vi "Autonomous Independent.vi"   [LabVIEW 2017]
doc: "This VI is called when autonomous begins, and will automatically be terminated when autonomous ends. You can carry out timed or sensor driven robot movement independently without needing to return to the caller."
uses:
  AutonActions.ctl
  WristPositions.ctl
  <vilib>/Rock Robotics/Network Tables/NT Write String.vi
  <vilib>/Rock Robotics/Network Tables/NT Read Number.vi
types:
  T1 = cluster{"TrgtCounts":i32, "CurrCounts":dbl, "SlowRng":dbl}
  T2 = cluster{"Heading":dbl, "Initial":dbl, "Range":dbl, "GyroSens":dbl}
  T3 = typedef "AutonActions.ctl" = enum16{"Initialize", "Stop", "Reset", "StraightForward", "StraightBack", "SolenoidControl", "TurnLeft90", "TurnRight90", "TurnLeft45", "TurnRight45", "PivotLeft90", "PivotRight90", "PivotLeft45", "PivotRight45", "PivotLeft30", "PivotRight30", "StraightForwardTime", "Release", "Shoot", "Wrist", "GripperToggle", "ElevUp", "ElevDown", "Pause", ""}
  T4 = typedef "WristPositions.ctl" = enum16{"MostDown", "AllDown", "MostUp", "AllUp"}
  T5 = cluster{"Action":T3, "DriveEncCnts":i32, "Accel?":bool, "Decel?":bool, "ElevEncCnts":i32, "Action2":T3, "Action2Trigger":i32, "WristPositions":T4, "SlowRng":dbl}[]
  T6 = cluster{"Action":T3, "DriveEncCnts":i32, "Accel?":bool, "Decel?":bool, "ElevEncCnts":i32, "Action2":T3, "Action2Trigger":i32, "WristPositions":T4, "SlowRng":dbl}
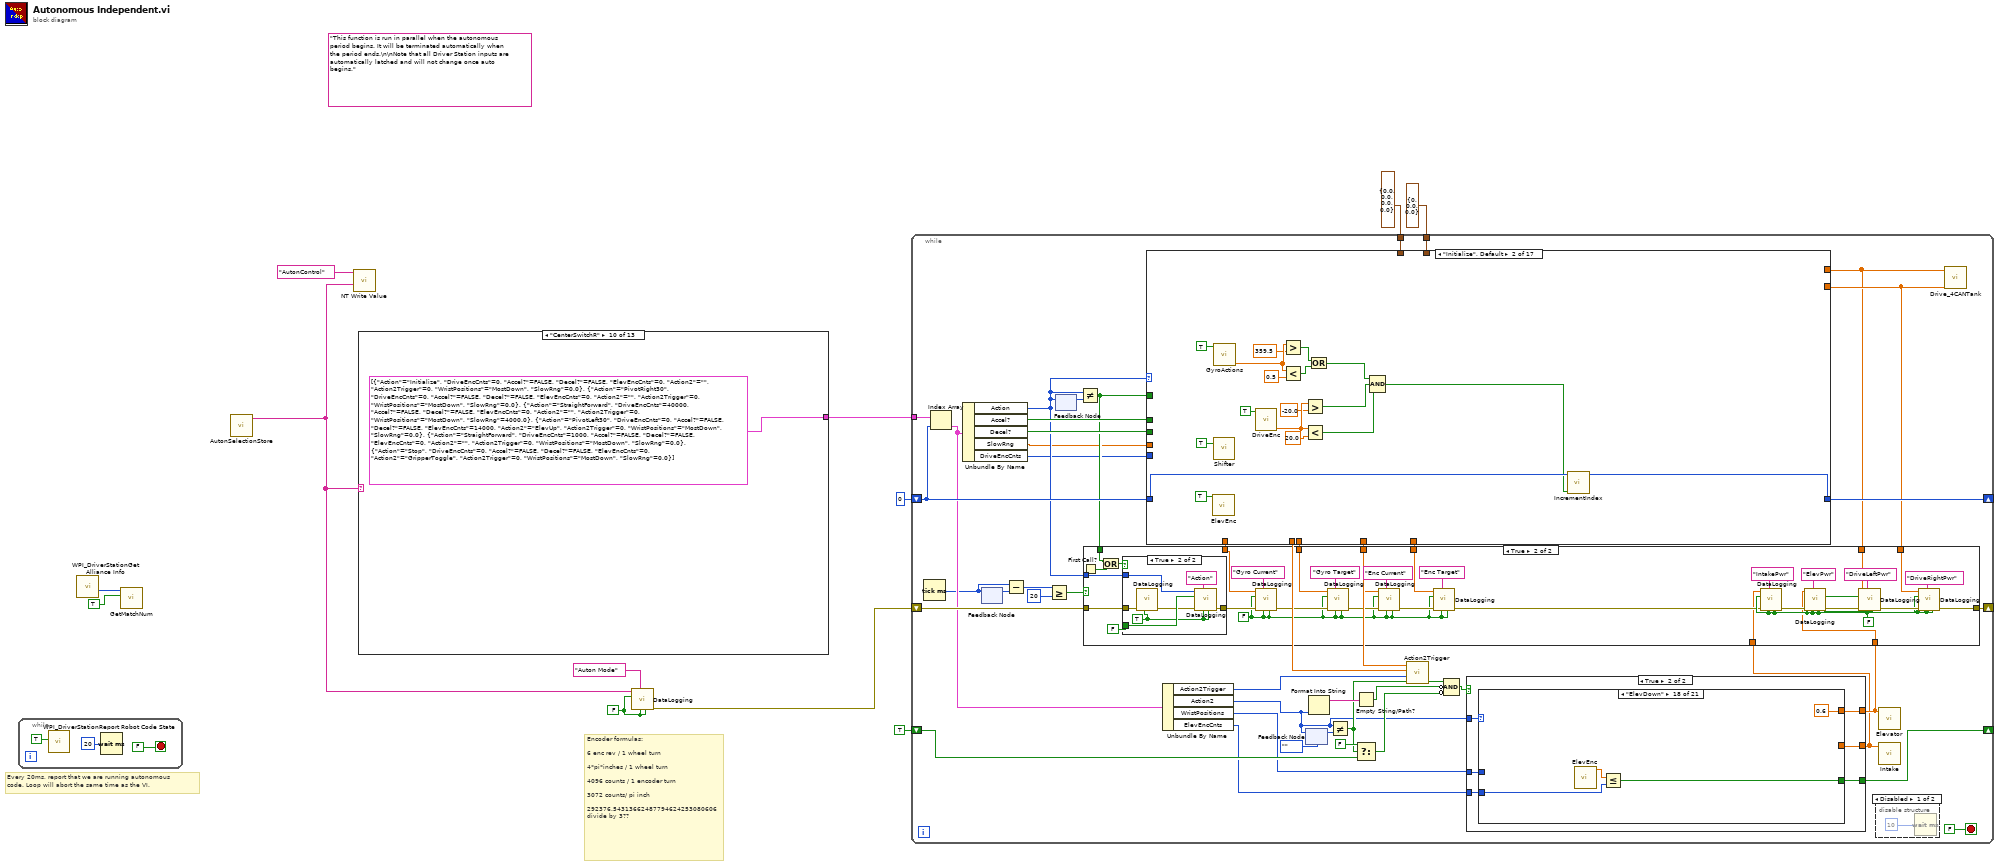
[diagram p0: block diagram]
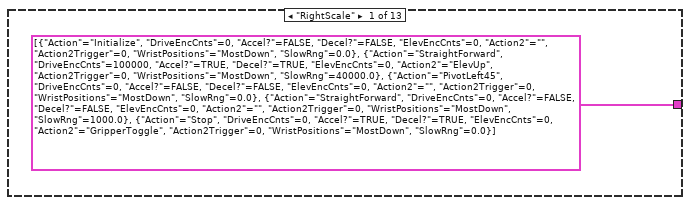
[diagram p2: hidden frame]
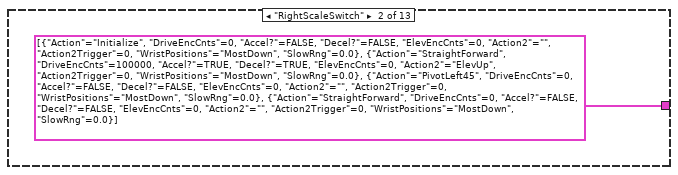
[diagram p3: hidden frame]
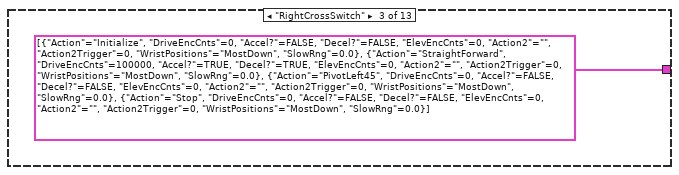
[diagram p4: hidden frame]
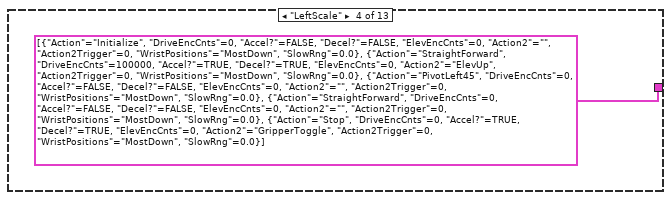
[diagram p5: hidden frame]
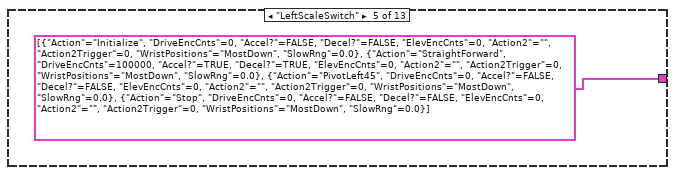
[diagram p6: hidden frame]
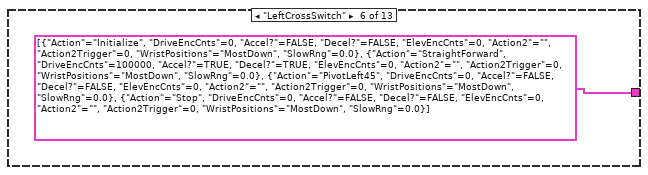
[diagram p7: hidden frame]
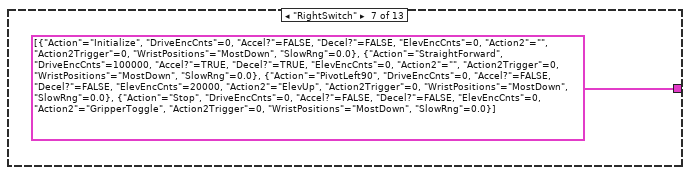
[diagram p8: hidden frame]
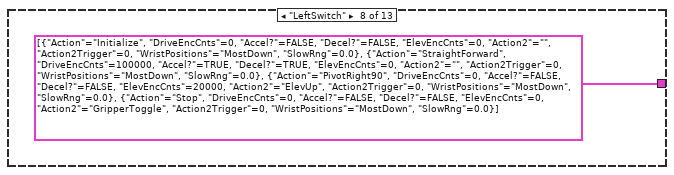
[diagram p9: hidden frame]
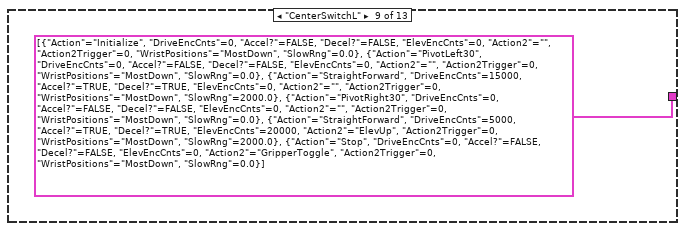
[diagram p10: hidden frame]
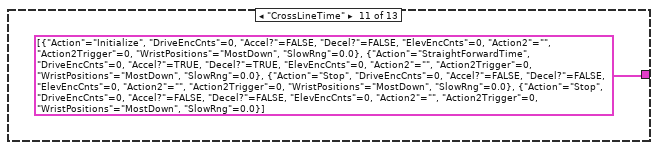
[diagram p11: hidden frame]
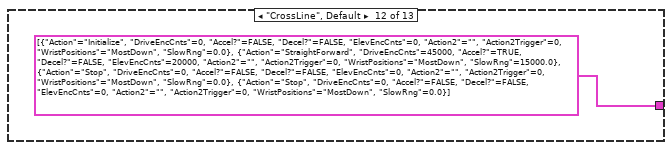
[diagram p12: hidden frame]
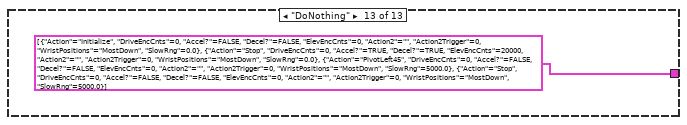
[diagram p13: hidden frame]
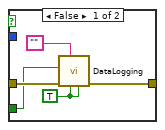
[diagram p15: hidden frame]
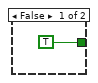
[diagram p16: hidden frame]
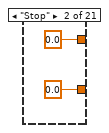
[diagram p18: hidden frame]
diagram:
  w7 = FALSE ("WriteToFile?")
  (unwired) "This function is run in parallel when the autonomous period begins. It will be terminated automatically when the period ends.\n\nNote that all Driver Station inputs are automatically latched and will not change once auto begins."
  # "Encoder formulas:\n\n6 enc rev / 1 wheel turn\n\n4*pi*inches / 1 wheel turn \n\n4096 counts / 1 encoder turn\n\n3072 counts/ pi inch\n\n292376.54313662487794624253080606\ndivide by 3??"
  # "Every 20ms, report that we are running autonomous\ncode. Loop will abort the same time as the VI."
  n1 = while {
    stop <- FALSE stop-if-true
    n2 = call <vilib>:"WPI_DriverStationReport Robot Code State.vi"("Autonomous"=TRUE) -> ()  [unwired: 10 in, 1 out]
    n3 = Wait (ms)(milliseconds to wait=u32 20) -> ()  [unwired: 1 out]
  }
  n4 = call <vilib>:"WPI_DriverStationGet Alliance Info.vi"() -> ("Match Number"=w6:u16)  [unwired: 11 out]
  n5 = call "GetMatchNum.vi"("Update?"=TRUE, "MatchNumberIn"=w6) -> ()  [unwired: 6 in, 1 out]
  n6 = call "AutonSelectionStore.vi"() -> ("AutonSelectionOut"=w1:string)  [unwired: 11 in]
  n7 = call-poly <vilib>:"NT Write Value.vi"("String"=w1, "Name"="AutonControl") -> ()  [unwired: 9 in, 1 out]
  n8 = case shown="\"CenterSwitchR\"" w1 {
    tunnel: [T5 [{"Action"=enum."Initialize", "DriveEncCnts"=0, "Accel?"=FALSE, "Decel?"=FALSE, "ElevEncCnts"=0, "Action2"=enum."", "Action2Trigger"=0, "WristPositions"=enum."MostDown", "SlowRng"=0.0}, {"Action"=enum."StraightForward", "DriveEncCnts"=100000, "Accel?"=TRUE, "Decel?"=TRUE, "ElevEncCnts"=0, "Action2"=enum."ElevUp", "Action2Trigger"=0, "WristPositions"=enum."MostDown", "SlowRng"=40000.0}, {"Action"=enum."PivotLeft45", "DriveEncCnts"=0, "Accel?"=FALSE, "Decel?"=FALSE, "ElevEncCnts"=0, "Action2"=enum."", "Action2Trigger"=0, "WristPositions"=enum."MostDown", "SlowRng"=0.0}, {"Action"=enum."StraightForward", "DriveEncCnts"=0, "Accel?"=FALSE, "Decel?"=FALSE, "ElevEncCnts"=0, "Action2"=enum."", "Action2Trigger"=0, "WristPositions"=enum."MostDown", "SlowRng"=1000.0}, {"Action"=enum."Stop", "DriveEncCnts"=0, "Accel?"=TRUE, "Decel?"=TRUE, "ElevEncCnts"=0, "Action2"=enum."GripperToggle", "Action2Trigger"=0, "WristPositions"=enum."MostDown", "SlowRng"=0.0}] T5 [{"Action"=enum."Initialize", "DriveEncCnts"=0, "Accel?"=FALSE, "Decel?"=FALSE, "ElevEncCnts"=0, "Action2"=enum."", "Action2Trigger"=0, "WristPositions"=enum."MostDown", "SlowRng"=0.0}, {"Action"=enum."StraightForward", "DriveEncCnts"=100000, "Accel?"=TRUE, "Decel?"=TRUE, "ElevEncCnts"=0, "Action2"=enum."ElevUp", "Action2Trigger"=0, "WristPositions"=enum."MostDown", "SlowRng"=0.0}, {"Action"=enum."PivotLeft45", "DriveEncCnts"=0, "Accel?"=FALSE, "Decel?"=FALSE, "ElevEncCnts"=0, "Action2"=enum."", "Action2Trigger"=0, "WristPositions"=enum."MostDown", "SlowRng"=0.0}, {"Action"=enum."StraightForward", "DriveEncCnts"=0, "Accel?"=FALSE, "Decel?"=FALSE, "ElevEncCnts"=0, "Action2"=enum."", "Action2Trigger"=0, "WristPositions"=enum."MostDown", "SlowRng"=0.0}] T5 [{"Action"=enum."Initialize", "DriveEncCnts"=0, "Accel?"=FALSE, "Decel?"=FALSE, "ElevEncCnts"=0, "Action2"=enum."", "Action2Trigger"=0, "WristPositions"=enum."MostDown", "SlowRng"=0.0}, {"Action"=enum."StraightForward", "DriveEncCnts"=100000, "Accel?"=TRUE, "Decel?"=TRUE, "ElevEncCnts"=0, "Action2"=enum."", "Action2Trigger"=0, "WristPositions"=enum."MostDown", "SlowRng"=0.0}, {"Action"=enum."PivotLeft45", "DriveEncCnts"=0, "Accel?"=FALSE, "Decel?"=FALSE, "ElevEncCnts"=0, "Action2"=enum."", "Action2Trigger"=0, "WristPositions"=enum."MostDown", "SlowRng"=0.0}, {"Action"=enum."Stop", "DriveEncCnts"=0, "Accel?"=FALSE, "Decel?"=FALSE, "ElevEncCnts"=0, "Action2"=enum."", "Action2Trigger"=0, "WristPositions"=enum."MostDown", "SlowRng"=0.0}] T5 [{"Action"=enum."Initialize", "DriveEncCnts"=0, "Accel?"=FALSE, "Decel?"=FALSE, "ElevEncCnts"=0, "Action2"=enum."", "Action2Trigger"=0, "WristPositions"=enum."MostDown", "SlowRng"=0.0}, {"Action"=enum."StraightForward", "DriveEncCnts"=100000, "Accel?"=TRUE, "Decel?"=TRUE, "ElevEncCnts"=0, "Action2"=enum."ElevUp", "Action2Trigger"=0, "WristPositions"=enum."MostDown", "SlowRng"=0.0}, {"Action"=enum."PivotLeft45", "DriveEncCnts"=0, "Accel?"=FALSE, "Decel?"=FALSE, "ElevEncCnts"=0, "Action2"=enum."", "Action2Trigger"=0, "WristPositions"=enum."MostDown", "SlowRng"=0.0}, {"Action"=enum."StraightForward", "DriveEncCnts"=0, "Accel?"=FALSE, "Decel?"=FALSE, "ElevEncCnts"=0, "Action2"=enum."", "Action2Trigger"=0, "WristPositions"=enum."MostDown", "SlowRng"=0.0}, {"Action"=enum."Stop", "DriveEncCnts"=0, "Accel?"=TRUE, "Decel?"=TRUE, "ElevEncCnts"=0, "Action2"=enum."GripperToggle", "Action2Trigger"=0, "WristPositions"=enum."MostDown", "SlowRng"=0.0}] T5 [{"Action"=enum."Initialize", "DriveEncCnts"=0, "Accel?"=FALSE, "Decel?"=FALSE, "ElevEncCnts"=0, "Action2"=enum."", "Action2Trigger"=0, "WristPositions"=enum."MostDown", "SlowRng"=0.0}, {"Action"=enum."StraightForward", "DriveEncCnts"=100000, "Accel?"=TRUE, "Decel?"=TRUE, "ElevEncCnts"=0, "Action2"=enum."", "Action2Trigger"=0, "WristPositions"=enum."MostDown", "SlowRng"=0.0}, {"Action"=enum."PivotLeft45", "DriveEncCnts"=0, "Accel?"=FALSE, "Decel?"=FALSE, "ElevEncCnts"=0, "Action2"=enum."", "Action2Trigger"=0, "WristPositions"=enum."MostDown", "SlowRng"=0.0}, {"Action"=enum."Stop", "DriveEncCnts"=0, "Accel?"=FALSE, "Decel?"=FALSE, "ElevEncCnts"=0, "Action2"=enum."", "Action2Trigger"=0, "WristPositions"=enum."MostDown", "SlowRng"=0.0}] T5 [{"Action"=enum."Initialize", "DriveEncCnts"=0, "Accel?"=FALSE, "Decel?"=FALSE, "ElevEncCnts"=0, "Action2"=enum."", "Action2Trigger"=0, "WristPositions"=enum."MostDown", "SlowRng"=0.0}, {"Action"=enum."StraightForward", "DriveEncCnts"=100000, "Accel?"=TRUE, "Decel?"=TRUE, "ElevEncCnts"=0, "Action2"=enum."", "Action2Trigger"=0, "WristPositions"=enum."MostDown", "SlowRng"=0.0}, {"Action"=enum."PivotLeft45", "DriveEncCnts"=0, "Accel?"=FALSE, "Decel?"=FALSE, "ElevEncCnts"=0, "Action2"=enum."", "Action2Trigger"=0, "WristPositions"=enum."MostDown", "SlowRng"=0.0}, {"Action"=enum."Stop", "DriveEncCnts"=0, "Accel?"=FALSE, "Decel?"=FALSE, "ElevEncCnts"=0, "Action2"=enum."", "Action2Trigger"=0, "WristPositions"=enum."MostDown", "SlowRng"=0.0}] T5 [{"Action"=enum."Initialize", "DriveEncCnts"=0, "Accel?"=FALSE, "Decel?"=FALSE, "ElevEncCnts"=0, "Action2"=enum."", "Action2Trigger"=0, "WristPositions"=enum."MostDown", "SlowRng"=0.0}, {"Action"=enum."StraightForward", "DriveEncCnts"=100000, "Accel?"=TRUE, "Decel?"=TRUE, "ElevEncCnts"=0, "Action2"=enum."", "Action2Trigger"=0, "WristPositions"=enum."MostDown", "SlowRng"=0.0}, {"Action"=enum."PivotLeft90", "DriveEncCnts"=0, "Accel?"=FALSE, "Decel?"=FALSE, "ElevEncCnts"=20000, "Action2"=enum."ElevUp", "Action2Trigger"=0, "WristPositions"=enum."MostDown", "SlowRng"=0.0}, {"Action"=enum."Stop", "DriveEncCnts"=0, "Accel?"=FALSE, "Decel?"=FALSE, "ElevEncCnts"=0, "Action2"=enum."GripperToggle", "Action2Trigger"=0, "WristPositions"=enum."MostDown", "SlowRng"=0.0}] T5 [{"Action"=enum."Initialize", "DriveEncCnts"=0, "Accel?"=FALSE, "Decel?"=FALSE, "ElevEncCnts"=0, "Action2"=enum."", "Action2Trigger"=0, "WristPositions"=enum."MostDown", "SlowRng"=0.0}, {"Action"=enum."StraightForward", "DriveEncCnts"=100000, "Accel?"=TRUE, "Decel?"=TRUE, "ElevEncCnts"=0, "Action2"=enum."", "Action2Trigger"=0, "WristPositions"=enum."MostDown", "SlowRng"=0.0}, {"Action"=enum."PivotRight90", "DriveEncCnts"=0, "Accel?"=FALSE, "Decel?"=FALSE, "ElevEncCnts"=20000, "Action2"=enum."ElevUp", "Action2Trigger"=0, "WristPositions"=enum."MostDown", "SlowRng"=0.0}, {"Action"=enum."Stop", "DriveEncCnts"=0, "Accel?"=FALSE, "Decel?"=FALSE, "ElevEncCnts"=0, "Action2"=enum."GripperToggle", "Action2Trigger"=0, "WristPositions"=enum."MostDown", "SlowRng"=0.0}] T5 [{"Action"=enum."Initialize", "DriveEncCnts"=0, "Accel?"=FALSE, "Decel?"=FALSE, "ElevEncCnts"=0, "Action2"=enum."", "Action2Trigger"=0, "WristPositions"=enum."MostDown", "SlowRng"=0.0}, {"Action"=enum."PivotLeft30", "DriveEncCnts"=0, "Accel?"=FALSE, "Decel?"=FALSE, "ElevEncCnts"=0, "Action2"=enum."", "Action2Trigger"=0, "WristPositions"=enum."MostDown", "SlowRng"=0.0}, {"Action"=enum."StraightForward", "DriveEncCnts"=15000, "Accel?"=TRUE, "Decel?"=TRUE, "ElevEncCnts"=0, "Action2"=enum."", "Action2Trigger"=0, "WristPositions"=enum."MostDown", "SlowRng"=2000.0}, {"Action"=enum."PivotRight30", "DriveEncCnts"=0, "Accel?"=FALSE, "Decel?"=FALSE, "ElevEncCnts"=0, "Action2"=enum."", "Action2Trigger"=0, "WristPositions"=enum."MostDown", "SlowRng"=0.0}, {"Action"=enum."StraightForward", "DriveEncCnts"=5000, "Accel?"=TRUE, "Decel?"=TRUE, "ElevEncCnts"=20000, "Action2"=enum."ElevUp", "Action2Trigger"=0, "WristPositions"=enum."MostDown", "SlowRng"=2000.0}, {"Action"=enum."Stop", "DriveEncCnts"=0, "Accel?"=FALSE, "Decel?"=FALSE, "ElevEncCnts"=0, "Action2"=enum."GripperToggle", "Action2Trigger"=0, "WristPositions"=enum."MostDown", "SlowRng"=0.0}] T5 [{"Action"=enum."Initialize", "DriveEncCnts"=0, "Accel?"=FALSE, "Decel?"=FALSE, "ElevEncCnts"=0, "Action2"=enum."", "Action2Trigger"=0, "WristPositions"=enum."MostDown", "SlowRng"=0.0}, {"Action"=enum."PivotRight30", "DriveEncCnts"=0, "Accel?"=FALSE, "Decel?"=FALSE, "ElevEncCnts"=0, "Action2"=enum."", "Action2Trigger"=0, "WristPositions"=enum."MostDown", "SlowRng"=0.0}, {"Action"=enum."StraightForward", "DriveEncCnts"=40000, "Accel?"=FALSE, "Decel?"=FALSE, "ElevEncCnts"=0, "Action2"=enum."", "Action2Trigger"=0, "WristPositions"=enum."MostDown", "SlowRng"=4000.0}, {"Action"=enum."PivotLeft30", "DriveEncCnts"=0, "Accel?"=FALSE, "Decel?"=FALSE, "ElevEncCnts"=14000, "Action2"=enum."ElevUp", "Action2Trigger"=0, "WristPositions"=enum."MostDown", "SlowRng"=0.0}, {"Action"=enum."StraightForward", "DriveEncCnts"=1000, "Accel?"=FALSE, "Decel?"=FALSE, "ElevEncCnts"=0, "Action2"=enum."", "Action2Trigger"=0, "WristPositions"=enum."MostDown", "SlowRng"=0.0}, {"Action"=enum."Stop", "DriveEncCnts"=0, "Accel?"=FALSE, "Decel?"=FALSE, "ElevEncCnts"=0, "Action2"=enum."GripperToggle", "Action2Trigger"=0, "WristPositions"=enum."MostDown", "SlowRng"=0.0}] T5 [{"Action"=enum."Initialize", "DriveEncCnts"=0, "Accel?"=FALSE, "Decel?"=FALSE, "ElevEncCnts"=0, "Action2"=enum."", "Action2Trigger"=0, "WristPositions"=enum."MostDown", "SlowRng"=0.0}, {"Action"=enum."StraightForwardTime", "DriveEncCnts"=0, "Accel?"=TRUE, "Decel?"=TRUE, "ElevEncCnts"=0, "Action2"=enum."", "Action2Trigger"=0, "WristPositions"=enum."MostDown", "SlowRng"=0.0}, {"Action"=enum."Stop", "DriveEncCnts"=0, "Accel?"=FALSE, "Decel?"=FALSE, "ElevEncCnts"=0, "Action2"=enum."", "Action2Trigger"=0, "WristPositions"=enum."MostDown", "SlowRng"=0.0}, {"Action"=enum."Stop", "DriveEncCnts"=0, "Accel?"=FALSE, "Decel?"=FALSE, "ElevEncCnts"=0, "Action2"=enum."", "Action2Trigger"=0, "WristPositions"=enum."MostDown", "SlowRng"=0.0}] T5 [{"Action"=enum."Initialize", "DriveEncCnts"=0, "Accel?"=FALSE, "Decel?"=FALSE, "ElevEncCnts"=0, "Action2"=enum."", "Action2Trigger"=0, "WristPositions"=enum."MostDown", "SlowRng"=0.0}, {"Action"=enum."StraightForward", "DriveEncCnts"=45000, "Accel?"=TRUE, "Decel?"=FALSE, "ElevEncCnts"=20000, "Action2"=enum."", "Action2Trigger"=0, "WristPositions"=enum."MostDown", "SlowRng"=15000.0}, {"Action"=enum."Stop", "DriveEncCnts"=0, "Accel?"=FALSE, "Decel?"=FALSE, "ElevEncCnts"=0, "Action2"=enum."", "Action2Trigger"=0, "WristPositions"=enum."MostDown", "SlowRng"=0.0}, {"Action"=enum."Stop", "DriveEncCnts"=0, "Accel?"=FALSE, "Decel?"=FALSE, "ElevEncCnts"=0, "Action2"=enum."", "Action2Trigger"=0, "WristPositions"=enum."MostDown", "SlowRng"=0.0}] T5 [{"Action"=enum."Initialize", "DriveEncCnts"=0, "Accel?"=FALSE, "Decel?"=FALSE, "ElevEncCnts"=0, "Action2"=enum."", "Action2Trigger"=0, "WristPositions"=enum."MostDown", "SlowRng"=0.0}, {"Action"=enum."Stop", "DriveEncCnts"=0, "Accel?"=TRUE, "Decel?"=TRUE, "ElevEncCnts"=20000, "Action2"=enum."", "Action2Trigger"=0, "WristPositions"=enum."MostDown", "SlowRng"=0.0}, {"Action"=enum."PivotLeft45", "DriveEncCnts"=0, "Accel?"=FALSE, "Decel?"=FALSE, "ElevEncCnts"=0, "Action2"=enum."", "Action2Trigger"=0, "WristPositions"=enum."MostDown", "SlowRng"=5000.0}, {"Action"=enum."Stop", "DriveEncCnts"=0, "Accel?"=FALSE, "Decel?"=FALSE, "ElevEncCnts"=0, "Action2"=enum."", "Action2Trigger"=0, "WristPositions"=enum."MostDown", "SlowRng"=5000.0}]] -> w12
    frame "RightScale" {
    }
    frame "RightScaleSwitch" {
    }
    frame "RightCrossSwitch" {
    }
    frame "LeftScale" {
    }
    frame "LeftScaleSwitch" {
    }
    frame "LeftCrossSwitch" {
    }
    frame "RightSwitch" {
    }
    frame "LeftSwitch" {
    }
    frame "CenterSwitchL" {
    }
    frame "CenterSwitchR" {
    }
    frame "CrossLineTime" {
    }
    frame "CrossLine", Default {
    }
    frame "DoNothing" {
    }
  }
  n9 = call "DataLogging.vi"("Tab?"=w7, "New Line?"=w7, "Name"="Auton Mode", "WriteToFile?"=w7, "Variant In"=w1) -> ("error out"=w8:errorcluster)  [unwired: 5 in, 1 out]
  n10 = while {
    tunnel: w12 -> [w73]
    shift-right: [w71] -> _
    shift-left: 0 ("IndexOut") -> [w72]
    tunnel: T2 {"Heading"=0.0, "Initial"=0.0, "Range"=0.0, "GyroSens"=0.0} ("GyroData") -> [w68]
    tunnel: T1 {"TrgtCounts"=0, "CurrCounts"=0.0, "SlowRng"=0.0} ("EncData") -> [w67]
    shift-right: [w58] -> _
    shift-left: w8 -> [w59]
    shift-right: [w48] -> _
    shift-left: TRUE -> [w53]
    stop <- FALSE stop-if-true
    n11 = Tick Count (ms)() -> (millisecond timer value=w33:u32)
    n12 = Index Array(array=w73, index=w72) -> (element=w41:T6)
    n13 = Unbundle By Name(w41) -> ("Action"=w56:T3, "Accel?"=w66:bool, "Decel?"=w65:bool, "SlowRng"=w36:dbl, "DriveEncCnts"=w47:i32)
    n14 = feedback-in #1(w33) -> ()
    n15 = feedback #1() -> (w32:u32)  [unwired: 1 in]
    n16 = Subtract(x=w33, y=w32) -> (x-y=w30:u32)
    n17 = Greater Or Equal?(x=w30, y=u32 20) -> (x >= y?=w31:bool)
    n18 = feedback-in #2(w56) -> ()
    n19 = feedback #2() -> (w70:T3)  [unwired: 1 in]
    n20 = Not Equal?(x=w56, y=w70) -> (x != y?=w57:bool)
    n21 = case shown="\"Initialize\", Default" w56 {
      tunnel: [w171 w198 w201 w216 w237 w251 w272 w279 w291 w313 w325 w331 w337 w351 w365 w378 w392] -> w71
      tunnel: w72 -> [w172 w199 w201 w209 w243 w252 w271 w278 w290 w312 w326 w332 w338 w352 w366 w379 w393]
      tunnel: w57 -> [w156 _ _ _ w227 w248 w263 w276 w288 w311 w316 w327 w336 w350 w364 w375 _]
      tunnel: [w176 _ w200 w217 w235 w254 w262 w284 w297 w302 w319 w328 w334 w348 w362 w377 w391] -> w60
      tunnel: [w168 _ w200 w217 w236 w253 w261 w285 w298 w301 w318 w328 w335 w349 w363 w376 w391] -> w61
      tunnel: w47 -> [w153 _ _ _ w233 _ _ _ _ _ _ _ _ _ _ _ _]
      tunnel: w66 -> [w165 _ _ _ w225 _ _ _ _ _ _ _ _ _ _ _ _]
      tunnel: w65 -> [w149 _ _ _ w226 _ _ _ _ _ _ _ _ _ _ _ _]
      tunnel: w68 -> [w164 _ _ _ w231 _ _ _ _ _ _ _ _ _ _ _ _]
      tunnel: w67 -> [w160 _ _ _ w229 _ _ _ _ _ _ _ _ _ _ _ _]
      tunnel: [w158 _ _ _ _ _ _ w273 _ w300 _ _ w333 w347 w361 _ _] -> w64
      tunnel: [w157 _ _ _ _ _ _ _ _ _ _ _ _ _ _ _ _] -> w63
      tunnel: [w155 _ _ _ _ _ _ _ _ _ _ _ _ _ _ _ _] -> w44
      tunnel: [w152 _ _ _ w219 _ _ _ _ _ _ _ _ _ _ _ _] -> w62
      tunnel: [w151 _ _ _ w232 _ _ _ _ _ _ _ _ _ _ _ _] -> w43
      tunnel: w36 -> [w147 _ _ _ _ _ _ _ _ _ _ _ _ _ _ _ _]
      frame "StraightForward" {
        w167 = -1.0  # MtrPwr
        w166 = 0.15  # MinPwr
        w162 = 0.25  # Range
        # "High Gear:  .000641"
        # "Low gear sensitivity = .00015"
        # "Negative\n= Forward"
        n22 = call "GyroActions.vi"() -> ("Fused Heading"=w158:dbl)  [unwired: 10 in, 1 out]
        n23 = Not(x=w156) -> (.not. x?=w173:bool)
        n24 = call "DriveEnc.vi"() -> ("RightEncder"=w155:dbl)  [unwired: 10 in, 1 out]
        n25 = call-poly <vilib>:"NT Read Value.vi"("Name"="StrtSens") -> ("Numeric"=w170:dbl)  [unwired: 9 in, 1 out]
        n26 = call "LockedHeading.vi"("LockHeading"=w173, "Heading In"=w158) -> ("LockedHeading"=w157:dbl)  [unwired: 7 in]
        n27 = feedback #3() -> (w154:dbl)  [unwired: 1 in]
        n28 = Select(t=w155, s=w156, f=w154) -> (s? t:f=w151:dbl)
        n29 = feedback-in #3(w151) -> ()
        n30 = disable-structure shown="Enabled" {
          disable-tunnel: [0.000641 ("Sensitivity") w178] -> w161
          disable-tunnel: w170 -> [_ w178]
          frame Enabled {
          }
          frame Disabled {
          }
        }
        n31 = Add(x=w153, y=w151) -> (x+y=w152:dbl)
        n32 = Greater Or Equal?(x=w155, y=w152) -> (x >= y?=w148:bool)
        n33 = Bundle By Name(cluster=w164, "GyroSens"=w161, "Heading"=w158, "Initial"=w157, "Range"=w162) -> (w163:T2)
        n34 = Bundle By Name(cluster=w160, "SlowRng"=w147, "CurrCounts"=w155, "TrgtCounts"=w152) -> (w159:T1)
        n35 = call "DriveStraight.vi"("EncData"=w159, "Decel?"=w149, "GyroData"=w163, "Accel?"=w165, "FirstTime?"=w156, "MinPwr"=w166, "MtrPwr"=w167) -> ("RightOut"=w175:dbl, "LeftOut"=w174:dbl)  [unwired: 3 in]
        n36 = And(x=w149, y=w148) -> (x .and. y?=w150:bool)
        n37 = call "IncrementIndex.vi"("Increment?"=w148, "IndexIn"=w172) -> ("IndexOut"=w171:i32)  [unwired: 9 in]
        n38 = case shown="False" w150 {
          tunnel: [w180 w181] -> w176
          tunnel: w174 -> [w180 _]
          tunnel: w175 -> [w179 _]
          tunnel: [w179 w181] -> w168
          frame False {
          }
          frame True {
            w181 = 0.0 ("Left")
          }
        }
      }
      frame "Initialize", Default {
        n39 = call "ElevEnc.vi"("Reset?"=TRUE) -> ()  [unwired: 10 in, 1 out]
        n40 = call "Shifter.vi"("Shift?"=TRUE) -> ()  [unwired: 3 in]
        n41 = call "GyroActions.vi"("Zero"=TRUE) -> ("Fused Heading"=w195:dbl)  [unwired: 9 in, 1 out]
        n42 = call "DriveEnc.vi"("Reset?"=TRUE) -> ("RightEncder"=w190:dbl)  [unwired: 9 in, 1 out]
        n43 = Greater?(x=w195, y=359.5 ("upper limit")) -> (0:w193:bool)
        n44 = Less?(x=w195, y=0.5 ("lower limit")) -> (x < y?=w196:bool)
        n45 = Greater?(x=w190, y=-20.0) -> (0:w186:bool)
        n46 = Less?(x=w190, y=20.0) -> (x < y?=w185:bool)
        n47 = Or(x=w193, y=w196) -> (x .or. y?=w187:bool)
        n48 = Compound Arithmetic op=AND(w187, w186, w185) -> (w184:bool)
        n49 = call "IncrementIndex.vi"("Increment?"=w184, "IndexIn"=w199) -> ("IndexOut"=w198:i32)  [unwired: 9 in]
      }
      frame "Stop" {
        w200 = 0.0 ("Left Motor Power")
      }
      frame "Reset" {
        w217 = 0.0 ("Left Motor Power")
        n50 = call "GyroActions.vi"("Zero"=TRUE) -> ("Fused Heading"=w207:dbl)  [unwired: 9 in, 1 out]
        n51 = call "DriveEnc.vi"("Reset?"=TRUE) -> ("RightEncder"=w213:dbl)  [unwired: 9 in, 1 out]
        n52 = Greater?(x=w207, y=359.5 ("upper limit")) -> (0:w208:bool)
        n53 = Less?(x=w207, y=0.5 ("lower limit")) -> (x < y?=w206:bool)
        n54 = In Range and Coerce(upper limit=100.0, x=w213, lower limit=-100.0) -> (In Range?=w214:bool)  [unwired: 1 out]
        n55 = Or(x=w208, y=w206) -> (x .or. y?=w202:bool)
        n56 = And(x=w202, y=w214) -> (x .and. y?=w215:bool)
        n57 = call "IncrementIndex.vi"("Increment?"=w215, "IndexIn"=w209) -> ("IndexOut"=w216:i32)  [unwired: 9 in]
      }
      frame "StraightBack" {
        n58 = call "DriveEnc.vi"() -> ("RightEncder"=w220:dbl)  [unwired: 10 in, 1 out]
        n59 = call "GyroActions.vi"("Update?"=FALSE) -> ("Fused Heading"=w228:dbl)  [unwired: 9 in, 1 out]
        n60 = Not(x=w227) -> (.not. x?=w240:bool)
        n61 = feedback #4() -> (w234:dbl)  [unwired: 1 in]
        n62 = Select(t=w220, s=w227, f=w234) -> (s? t:f=w232:dbl)
        n63 = feedback-in #4(w232) -> ()
        n64 = call "LockedHeading.vi"("LockHeading"=w240, "Heading In"=w228) -> ("LockedHeading"=w222:dbl)  [unwired: 7 in]
        n65 = Add(x=w233, y=w232) -> (x+y=w219:dbl)
        n66 = Greater Or Equal?(x=w220, y=w219) -> (x >= y?=w238:bool)
        n67 = Bundle By Name(cluster=w231, "GyroSens"=0.000641, "Heading"=w228, "Initial"=w222, "Range"=0.25) -> (w230:T2)
        n68 = Bundle By Name(cluster=w229, "SlowRng"=40000.0, "CurrCounts"=w220, "TrgtCounts"=w219) -> (w224:T1)
        n69 = call "DriveStraight.vi"("EncData"=w224, "Decel?"=w226, "GyroData"=w230, "Accel?"=w225, "FirstTime?"=w227, "MinPwr"=w222, "MtrPwr"=w228) -> ("RightOut"=w242:dbl, "LeftOut"=w241:dbl)  [unwired: 3 in]
        n70 = case shown="True" w238 {
          tunnel: [w245 w246] -> w235
          tunnel: w241 -> [w245 _]
          tunnel: w242 -> [w244 _]
          tunnel: [w244 w246] -> w236
          frame False {
          }
          frame True {
            w246 = 0.0 ("Left")
          }
        }
        n71 = call "IncrementIndex.vi"("Increment?"=w238, "IndexIn"=w243) -> ("IndexOut"=w237:i32)  [unwired: 9 in]
      }
      frame "TurnLeft90" {
        w249 = -90.0  # Dir&Deg
        w256 = 65.0  # Slow Range
        w257 = 1.0  # Motor Power In
        w259 = 0.25  # Target Range
        w258 = 0.24  # Min Power
        n72 = call "GyroActions.vi"() -> ("Fused Heading"=w255:dbl)  [unwired: 10 in, 1 out]
        n73 = call "TurnSmooth.vi"("Pivot"=FALSE, "Min Power"=w258, "FirstTime?"=w248, "Target Range"=w259, "Current Position"=w255, "Dir&Deg"=w249, "Slow Range"=w256, "Motor Power In"=w257) -> ("Done"=w250:bool, "Right Motor Power"=w253:dbl, "Left Motor Power"=w254:dbl)  [unwired: 1 out]
        n74 = call "IncrementIndex.vi"("Increment?"=w250, "IndexIn"=w252) -> ("IndexOut"=w251:i32)  [unwired: 9 in]
      }
      frame "TurnRight90" {
        w268 = 90.0  # Dir&Deg
        w267 = 65.0  # Slow Range
        w266 = 1.0  # Motor Power In
        w269 = 0.25  # Target Range
        w260 = 0.24  # Min Power
        n75 = call "GyroActions.vi"() -> ("Fused Heading"=w264:dbl)  [unwired: 10 in, 1 out]
        n76 = call "TurnSmooth.vi"("Pivot"=FALSE, "Min Power"=w260, "FirstTime?"=w263, "Target Range"=w269, "Current Position"=w264, "Dir&Deg"=w268, "Slow Range"=w267, "Motor Power In"=w266) -> ("Done"=w265:bool, "Right Motor Power"=w261:dbl, "Left Motor Power"=w262:dbl)  [unwired: 1 out]
        n77 = call "IncrementIndex.vi"("Increment?"=w265, "IndexIn"=w271) -> ("IndexOut"=w272:i32)  [unwired: 9 in]
      }
      frame "TurnLeft45" {
        w275 = -45.0  # Dir&Deg
        w280 = 65.0  # Slow Range
        w281 = 1.0  # Motor Power In
        w282 = 0.25  # Target Range
        w283 = 0.24  # Min Power
        n78 = call "GyroActions.vi"() -> ("Fused Heading"=w274:dbl)  [unwired: 10 in, 1 out]
        n79 = call "TurnSmooth.vi"("Pivot"=FALSE, "Min Power"=w283, "FirstTime?"=w276, "Target Range"=w282, "Current Position"=w274, "Dir&Deg"=w275, "Slow Range"=w280, "Motor Power In"=w281) -> ("Done"=w286:bool, "DegToTarget"=w273:dbl, "Right Motor Power"=w285:dbl, "Left Motor Power"=w284:dbl)
        n80 = call "IncrementIndex.vi"("Increment?"=w286, "IndexIn"=w278) -> ("IndexOut"=w279:i32)  [unwired: 9 in]
      }
      frame "TurnRight45" {
        w287 = 45.0  # Dir&Deg
        w292 = 65.0  # Slow Range
        w293 = 1.0  # Motor Power In
        w294 = 0.25  # Target Range
        w295 = 0.24  # Min Power
        n81 = call "GyroActions.vi"() -> ("Fused Heading"=w296:dbl)  [unwired: 10 in, 1 out]
        n82 = call "TurnSmooth.vi"("Pivot"=FALSE, "Min Power"=w295, "FirstTime?"=w288, "Target Range"=w294, "Current Position"=w296, "Dir&Deg"=w287, "Slow Range"=w292, "Motor Power In"=w293) -> ("Done"=w299:bool, "Right Motor Power"=w298:dbl, "Left Motor Power"=w297:dbl)  [unwired: 1 out]
        n83 = call "IncrementIndex.vi"("Increment?"=w299, "IndexIn"=w290) -> ("IndexOut"=w291:i32)  [unwired: 9 in]
      }
      frame "PivotLeft90" {
        w303 = 0.3  # Min Power
        w304 = 0.25  # Target Range
        w305 = 1.0  # Motor Power In
        w306 = 4.0  # Slow Range
        w308 = -90.0  # Dir&Deg
        n84 = call "GyroActions.vi"() -> ("Fused Heading"=w307:dbl)  [unwired: 10 in, 1 out]
        n85 = call "TurnSmooth.vi"("Pivot"=TRUE ("PivotDir"), "Min Power"=w303, "FirstTime?"=w311, "Target Range"=w304, "Current Position"=w307, "Dir&Deg"=w308, "Slow Range"=w306, "Motor Power In"=w305) -> ("Done"=w310:bool, "DegToTarget"=w300:dbl, "Right Motor Power"=w301:dbl, "Left Motor Power"=w302:dbl)
        n86 = call "IncrementIndex.vi"("Increment?"=w310, "IndexIn"=w312) -> ("IndexOut"=w313:i32)  [unwired: 9 in]
      }
      frame "PivotRight90" {
        w317 = 0.3  # Min Power
        w323 = 0.25  # Target Range
        w320 = 1.0  # Motor Power In
        w321 = 4.0  # Slow Range
        w322 = 90.0  # Dir&Deg
        n87 = call "GyroActions.vi"() -> ("Fused Heading"=w324:dbl)  [unwired: 10 in, 1 out]
        n88 = call "TurnSmooth.vi"("Pivot"=TRUE ("PivotDir"), "Min Power"=w317, "FirstTime?"=w316, "Target Range"=w323, "Current Position"=w324, "Dir&Deg"=w322, "Slow Range"=w321, "Motor Power In"=w320) -> ("Done"=w314:bool, "Right Motor Power"=w318:dbl, "Left Motor Power"=w319:dbl)  [unwired: 1 out]
        n89 = call "IncrementIndex.vi"("Increment?"=w314, "IndexIn"=w326) -> ("IndexOut"=w325:i32)  [unwired: 9 in]
      }
      frame "Pause" {
        w328 = 0.0 ("Left Motor Power")
        n90 = call "Wait.vi"("Target Time (s)"=0.75, "First Time?"=w327) -> ("Completed"=w330:bool)  [unwired: 8 in, 1 out]
        n91 = call "IncrementIndex.vi"("Increment?"=w330, "IndexIn"=w332) -> ("IndexOut"=w331:i32)  [unwired: 9 in]
      }
      frame "PivotLeft45" {
        w343 = 0.18  # Min Power
        w342 = 0.25  # Target Range
        w339 = 1.0  # Motor Power In
        w340 = 30.0  # Slow Range
        w341 = -45.0  # Dir&Deg
        n92 = call "GyroActions.vi"() -> ("Fused Heading"=w345:dbl)  [unwired: 10 in, 1 out]
        n93 = call "TurnSmooth.vi"("Pivot"=TRUE ("PivotDir"), "Min Power"=w343, "FirstTime?"=w336, "Target Range"=w342, "Current Position"=w345, "Dir&Deg"=w341, "Slow Range"=w340, "Motor Power In"=w339) -> ("Done"=w346:bool, "DegToTarget"=w333:dbl, "Right Motor Power"=w335:dbl, "Left Motor Power"=w334:dbl)
        n94 = call "IncrementIndex.vi"("Increment?"=w346, "IndexIn"=w338) -> ("IndexOut"=w337:i32)  [unwired: 9 in]
      }
      frame "PivotLeft30" {
        w357 = 0.18  # Min Power
        w356 = 0.25  # Target Range
        w353 = 1.0  # Motor Power In
        w354 = 20.0  # Slow Range
        w355 = -30.0  # Dir&Deg
        n95 = call "GyroActions.vi"() -> ("Fused Heading"=w359:dbl)  [unwired: 10 in, 1 out]
        n96 = call "TurnSmooth.vi"("Pivot"=TRUE ("PivotDir"), "Min Power"=w357, "FirstTime?"=w350, "Target Range"=w356, "Current Position"=w359, "Dir&Deg"=w355, "Slow Range"=w354, "Motor Power In"=w353) -> ("Done"=w360:bool, "DegToTarget"=w347:dbl, "Right Motor Power"=w349:dbl, "Left Motor Power"=w348:dbl)
        n97 = call "IncrementIndex.vi"("Increment?"=w360, "IndexIn"=w352) -> ("IndexOut"=w351:i32)  [unwired: 9 in]
      }
      frame "PivotRight30" {
        w371 = 0.18  # Min Power
        w370 = 0.5  # Target Range
        w367 = 1.0  # Motor Power In
        w368 = 20.0  # Slow Range
        w369 = 30.0  # Dir&Deg
        n98 = call "GyroActions.vi"() -> ("Fused Heading"=w373:dbl)  [unwired: 10 in, 1 out]
        n99 = call "TurnSmooth.vi"("Pivot"=TRUE ("PivotDir"), "Min Power"=w371, "FirstTime?"=w364, "Target Range"=w370, "Current Position"=w373, "Dir&Deg"=w369, "Slow Range"=w368, "Motor Power In"=w367) -> ("Done"=w374:bool, "DegToTarget"=w361:dbl, "Right Motor Power"=w363:dbl, "Left Motor Power"=w362:dbl)
        n100 = call "IncrementIndex.vi"("Increment?"=w374, "IndexIn"=w366) -> ("IndexOut"=w365:i32)  [unwired: 9 in]
      }
      frame "PivotRight45" {
        w384 = 0.3  # Min Power
        w383 = 0.25  # Target Range
        w380 = 1.0  # Motor Power In
        w381 = 4.0  # Slow Range
        w382 = 45.0  # Dir&Deg
        n101 = call "GyroActions.vi"() -> ("Fused Heading"=w386:dbl)  [unwired: 10 in, 1 out]
        n102 = call "TurnSmooth.vi"("Pivot"=TRUE ("PivotDir"), "Min Power"=w384, "FirstTime?"=w375, "Target Range"=w383, "Current Position"=w386, "Dir&Deg"=w382, "Slow Range"=w381, "Motor Power In"=w380) -> ("Done"=w387:bool, "Right Motor Power"=w376:dbl, "Left Motor Power"=w377:dbl)  [unwired: 1 out]
        n103 = call "IncrementIndex.vi"("Increment?"=w387, "IndexIn"=w379) -> ("IndexOut"=w378:i32)  [unwired: 9 in]
      }
      frame "StraightForwardTime" {
        n104 = call "Wait.vi"("Target Time (s)"=1.0, "First Time?"=TRUE) -> ("Completed"=w390:bool)  [unwired: 8 in, 1 out]
        n105 = Select(t=0.0, s=w390, f=1.0) -> (s? t:f=w391:dbl)
        n106 = call "IncrementIndex.vi"("Increment?"=w390, "IndexIn"=w393) -> ("IndexOut"=w392:i32)  [unwired: 9 in]
      }
    }
    n107 = Unbundle By Name(w41) -> ("Action2Trigger"=w39:i32, "Action2"=w40:T3, "WristPositions"=w38:T4, "ElevEncCnts"=w37:i32)
    n108 = feedback #5(AutonActions."" ("Action2")) -> (w54:T3)
    n109 = feedback-in #5(w40) -> ()
    n110 = Format Into String(w40) -> (resulting string=w55:string)  [unwired: 3 in, 1 out]
    n111 = Not Equal?(x=w40, y=w54) -> (x != y?=w45:bool)
    n112 = Empty String/Path?(string/path=w55) -> (empty?=w42:bool)
    n113 = Select(t=FALSE, s=w45, f=w53) -> (s? t:f=w51:bool)
    n114 = call "Action2Trigger.vi"("NewAction?"=w45, "Target"=w39, "Enc Initial"=w43, "Current"=w44) -> ("Triggered"=w46:bool)  [unwired: 7 in]
    n115 = Compound Arithmetic op=AND(w46, invert w42, invert w51) -> (w49:bool)
    n116 = case shown="True" w49 {
      tunnel: [TRUE w123] -> w48
      tunnel: w40 -> [_ w126]
      tunnel: [_ w125] -> w35
      tunnel: [_ w124] -> w34
      tunnel: w38 -> [_ w122]
      tunnel: w37 -> [_ w121]
      frame False {
      }
      frame True {
        n117 = case shown="\"ElevDown\"" w126 {
          tunnel: [_ 0.0 _ _ _ _ _ _ _ _ _ _ _ _ _ _ -0.85 ("Left Motor Power") 0.6 ("Left Motor Power") _ _ _] -> w125
          tunnel: [_ 0.0 _ _ _ _ _ _ _ _ _ _ _ _ 0.4 ("Left Motor Power") 1.0 ("Left Motor Power") _ _ _ _ _] -> w124
          tunnel: [_ _ _ _ _ _ _ _ _ _ _ _ _ _ _ _ w133 w137 _ TRUE ("Grip") w145] -> w123
          tunnel: w122 -> [_ _ _ _ _ _ _ _ _ _ _ _ _ _ _ _ _ _ _ w140 _]
          tunnel: w121 -> [_ _ _ _ _ _ _ _ _ _ _ _ _ _ _ _ w132 w136 _ _ _]
          frame "Initialize", Default {
          }
          frame "Stop" {
          }
          frame "Reset" {
          }
          frame "StraightForward" {
          }
          frame "StraightBack" {
          }
          frame "SolenoidControl" {
          }
          frame "TurnLeft90" {
          }
          frame "TurnRight90" {
          }
          frame "TurnLeft45" {
          }
          frame "TurnRight45" {
          }
          frame "PivotLeft90" {
          }
          frame "PivotRight90" {
          }
          frame "PivotLeft45" {
          }
          frame "PivotRight45" {
          }
          frame "Release" {
          }
          frame "Shoot" {
          }
          frame "ElevUp" {
            n118 = call "ElevEnc.vi"() -> ("ElevEnc"=w131:dbl)  [unwired: 11 in]
            n119 = Greater Or Equal?(x=w131, y=w132) -> (x >= y?=w133:bool)
          }
          frame "ElevDown" {
            n120 = call "ElevEnc.vi"() -> ("ElevEnc"=w135:dbl)  [unwired: 11 in]
            n121 = Less Or Equal?(x=w135, y=w136) -> (x <= y?=w137:bool)
          }
          frame "Pause" {
          }
          frame "Wrist" {
            n122 = case shown="\"AllDown\"" w140 {
              frame "MostDown", Default {
                n123 = call "Wrist.vi"("MostDown"=TRUE) -> ()  [unwired: 7 in]
              }
              frame "AllDown" {
                n124 = call "Wrist.vi"("AllDown"=TRUE) -> ()  [unwired: 7 in]
              }
              frame "MostUp" {
                n125 = call "Wrist.vi"("MostUp"=TRUE) -> ()  [unwired: 7 in]
              }
              frame "AllUp" {
                n126 = call "Wrist.vi"("AllUp"=TRUE) -> ()  [unwired: 7 in]
              }
            }
          }
          frame "GripperToggle" {
            w145 = TRUE ("Grip")
            n127 = call "Gripper.vi"("Grip"=w145) -> ()  [unwired: 3 in]
          }
        }
      }
    }
    n128 = case shown="True" w31 {
      tunnel: w64 -> [_ w105]
      tunnel: w63 -> [_ w102]
      tunnel: w62 -> [_ w97]
      tunnel: w61 -> [_ w92]
      tunnel: w60 -> [_ w91]
      tunnel: w59 -> [w74 w88]
      tunnel: [w74 w87] -> w58
      tunnel: w57 -> [_ w81]
      tunnel: w56 -> [_ w79]
      tunnel: w44 -> [_ w77]
      tunnel: w35 -> [_ w76]
      tunnel: w34 -> [_ w75]
      frame False {
      }
      frame True {
        w86 = FALSE ("New Line?")
        w80 = FALSE ("New Line?")
        n129 = First Call?() -> (First Call?: T/F=w83:bool)
        n130 = Or(x=w81, y=w83) -> (x .or. y?=w84:bool)
        n131 = case shown="True" w84 {
          tunnel: w79 -> [_ w118]
          tunnel: [w111 w117] -> w106
          tunnel: w88 -> [w110 w114]
          tunnel: FALSE ("WriteToFile?") -> [w108 w116]
          frame False {
            w109 = TRUE ("Tab?")
            n132 = call "DataLogging.vi"("Tab?"=w109, "New Line?"=w109, "Name"="", "error in (no error)"=w110, "WriteToFile?"=w108) -> ("error out"=w111:errorcluster)  [unwired: 5 in, 1 out]
          }
          frame True {
            w115 = TRUE ("New Line?")
            n133 = call "DataLogging.vi"("New Line?"=w115, "error in (no error)"=w114) -> ("error out"=w113:errorcluster)  [unwired: 8 in, 1 out]
            n134 = call "DataLogging.vi"("Tab?"=w115, "New Line?"=w115, "Name"="Action", "error in (no error)"=w113, "WriteToFile?"=w116, "Variant In"=w118) -> ("error out"=w117:errorcluster)  [unwired: 4 in, 1 out]
          }
        }
        n135 = call "DataLogging.vi"("Tab?"=w80, "New Line?"=w80, "Name"="Gyro Current", "error in (no error)"=w106, "WriteToFile?"=w80, "Variant In"=w105) -> ("error out"=w103:errorcluster)  [unwired: 4 in, 1 out]
        n136 = call "DataLogging.vi"("Tab?"=w80, "New Line?"=w80, "Name"="Gyro Target", "error in (no error)"=w103, "WriteToFile?"=w80, "Variant In"=w102) -> ("error out"=w99:errorcluster)  [unwired: 4 in, 1 out]
        n137 = call "DataLogging.vi"("Tab?"=w80, "New Line?"=w80, "Name"="Enc Current", "error in (no error)"=w99, "WriteToFile?"=w80, "Variant In"=w77) -> ("error out"=w98:errorcluster)  [unwired: 4 in, 1 out]
        n138 = call "DataLogging.vi"("Tab?"=w80, "New Line?"=w80, "Name"="Enc Target", "error in (no error)"=w98, "WriteToFile?"=w80, "Variant In"=w97) -> ("error out"=w78:errorcluster)  [unwired: 4 in, 1 out]
        n139 = call "DataLogging.vi"("Tab?"=w86, "New Line?"=w86, "Name"="IntakePwr", "error in (no error)"=w78, "WriteToFile?"=w86, "Variant In"=w75) -> ("error out"=w82:errorcluster)  [unwired: 4 in, 1 out]
        n140 = call "DataLogging.vi"("Tab?"=w86, "New Line?"=w86, "Name"="ElevPwr", "error in (no error)"=w82, "WriteToFile?"=w86, "Variant In"=w76) -> ("error out"=w90:errorcluster)  [unwired: 4 in, 1 out]
        n141 = call "DataLogging.vi"("Tab?"=w86, "New Line?"=w86, "Name"="DriveLeftPwr", "error in (no error)"=w90, "WriteToFile?"=w86, "Variant In"=w91) -> ("error out"=w89:errorcluster)  [unwired: 4 in, 1 out]
        n142 = call "DataLogging.vi"("Tab?"=w86, "New Line?"=w86, "Name"="DriveRightPwr", "error in (no error)"=w89, "WriteToFile?"=w86, "Variant In"=w92) -> ("error out"=w87:errorcluster)  [unwired: 4 in, 1 out]
      }
    }
    n143 = disable-structure shown="Disabled" {
      frame Disabled {
        n144 = Wait (ms)(milliseconds to wait=u32 10) -> ()  [unwired: 1 out]
      }
      frame Enabled {
      }
    }
    n145 = call "Elevator.vi"("Power"=w35) -> ()  [unwired: 11 in]
    n146 = call "Intake.vi"("Power"=w34) -> ()  [unwired: 11 in]
    n147 = call "Drive_4CANTank.vi"("RightMotor"=w61, "LeftMotor"=w60) -> ()  [unwired: 10 in]
  }
